vi "EventLoop 2.vi"() -> ()   [LabVIEW 2017, in "tmpevent.lvlib"]
uses:
  tmpevent.lvlib
  Communication/QueueRepo.Action.ctl
  Communication/Communication.lvlib
panel:
  out "Data 2":variant
  out "current time":timestamp
  out "Data":variant
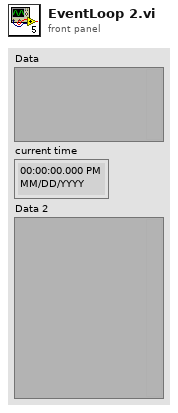
[diagram p1: front panel]
types:
  T1 = typedef "Communication.lvlib/QueueRepo.Action.ctl" = enum16{"Add", "Get", "Destroy", "Get All", "Clear"}
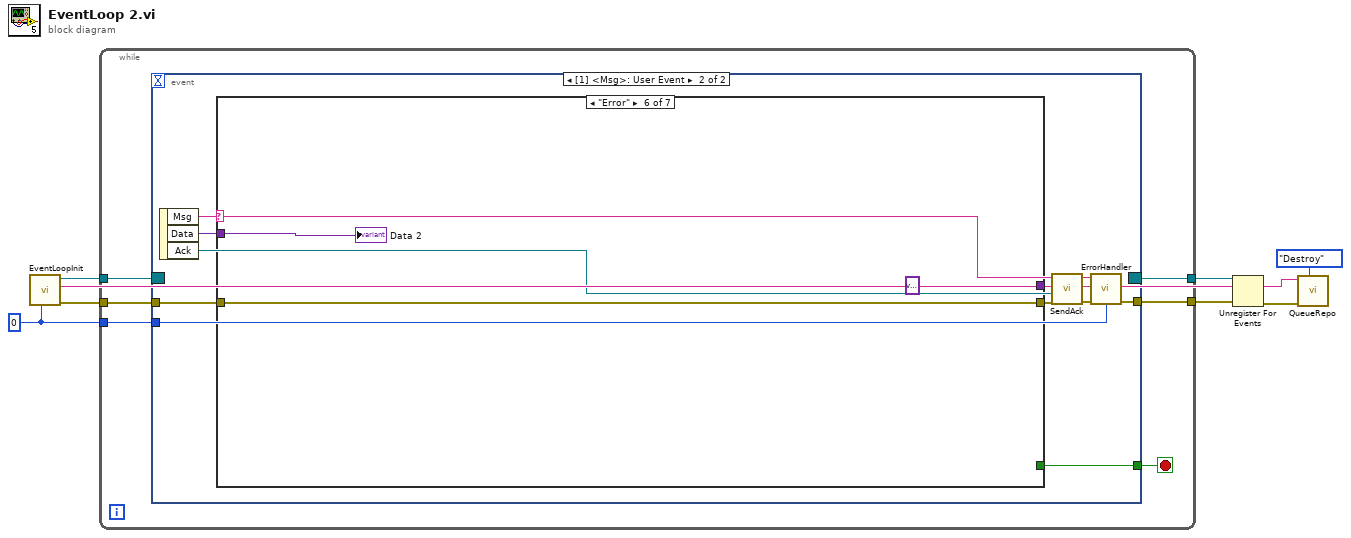
[diagram p0: block diagram]
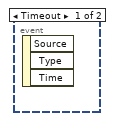
[diagram p2: hidden frame]
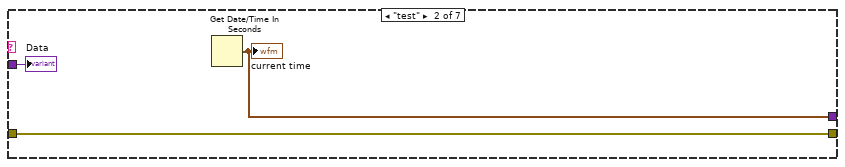
[diagram p4: hidden frame]
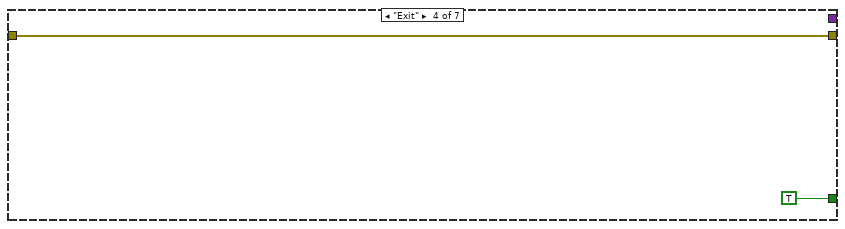
[diagram p6: hidden frame]
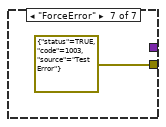
[diagram p8: hidden frame]
diagram:
  w6 = 0 ("Instance")
  n1 = call "EventLoopInit.vi"("Instance"=w6) -> ("error out"=w7:errorcluster, "Loop Name"=w3:string, "Event Registration Refnum"=w8:refnum<event-registration>)  [unwired: 8 in]
  n2 = while {
    tunnel: w8 -> [w14]
    tunnel: w7 -> [w13]
    tunnel: w6 -> [w12]
    tunnel: [w10] -> w5
    tunnel: [w9] -> w4
    stop <- w11 stop-if-true
    n3 = event shown="[1] <Msg>: User Event" {
      selector: w14 -> [_ _]
      dyn-events: [_ _] -> w10
      timeout: _ -> [_ _]
      tunnel: w13 -> [_ w23]
      tunnel: [_ w19] -> w9
      tunnel: w12 -> [_ w18]
      tunnel: [_ w15] -> w11
      event Timeout {
        n4 = event-data() -> ()  [unwired: 1 in, 3 out]
      }
      event User Event {
        n5 = event-data() -> ("Msg"=w20:string, "Data"=w24:variant, "Ack"=w22:refnum<notifier>)  [unwired: 1 in]
        n6 = case shown="\"Error\"" w20 {
          tunnel: w24 -> [_ w27 _ _ _ w33 _]
          tunnel: w23 -> [w25 w28 w29 w31 w32 w34 _]
          tunnel: [_ w26 _ _ _ variant _] -> w17
          tunnel: [w25 w28 w29 w31 w32 w34 errorcluster {"status"=TRUE, "code"=1003, "source"="Test Error"} ("error out")] -> w16
          tunnel: [_ _ _ TRUE _ _ _] -> w15
          frame Default {
          }
          frame "test" {
            n7 = Get Date/Time In Seconds() -> (seconds since 1Jan1904=w26:timestamp)
            "current time" <- w26
            "Data" <- w27
          }
          frame "Init" {
          }
          frame "Exit" {
          }
          frame "Tick" {
          }
          frame "Error" {
            "Data 2" <- w33
          }
          frame "ForceError" {
          }
        }
        n8 = call "SendAck.vi"("error in (no error)"=w16, "Ack"=w22, "Variant"=w17) -> ("error out"=w21:errorcluster)  [unwired: 8 in]
        n9 = call "ErrorHandler.vi"("Instance"=w18, "error in (no error)"=w21, "Msg"=w20) -> ("error out"=w19:errorcluster)  [unwired: 8 in]
      }
    }
  }
  n10 = Unregister For Events(event registration refnum=w5, error in=w4) -> (error out=w2:errorcluster)
  n11 = call "QueueRepo.vi"("Action"=QueueRepo.Action."Destroy", "error in (no error)"=w2, "Name"=w3) -> ()  [unwired: 5 in, 4 out]
